vi "Build Tree.vi"(8 "Actual Path":path[](array[path]), 10 "Expected Path":path[](array[path]), 11 "Tree Refnum":refnum<vi>) -> ()   [LabVIEW 2023]
doc: "Populates the tree control identified by <B>Tree Refnum</B> with the other inputs, highlighting each row appropriately."
uses:
  11d6df90-a5f7-4652-ac9b-e2f8193509e9.vi
  <userlib>/_OpenG.lib/file/file.llb/Strip Path - Arrays__ogtk.vi
  <userlib>/_OpenG.lib/array/array.llb/Filter 1D Array with Scalar (Path)__ogtk.vi
  <userlib>/_OpenG.lib/file/file.llb/openg_file.lvlib
  <userlib>/_OpenG.lib/array/array.llb/openg_array.lvlib
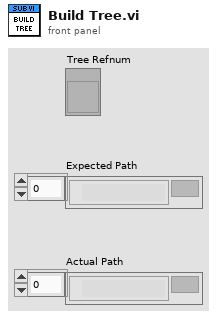
[diagram p1: front panel]
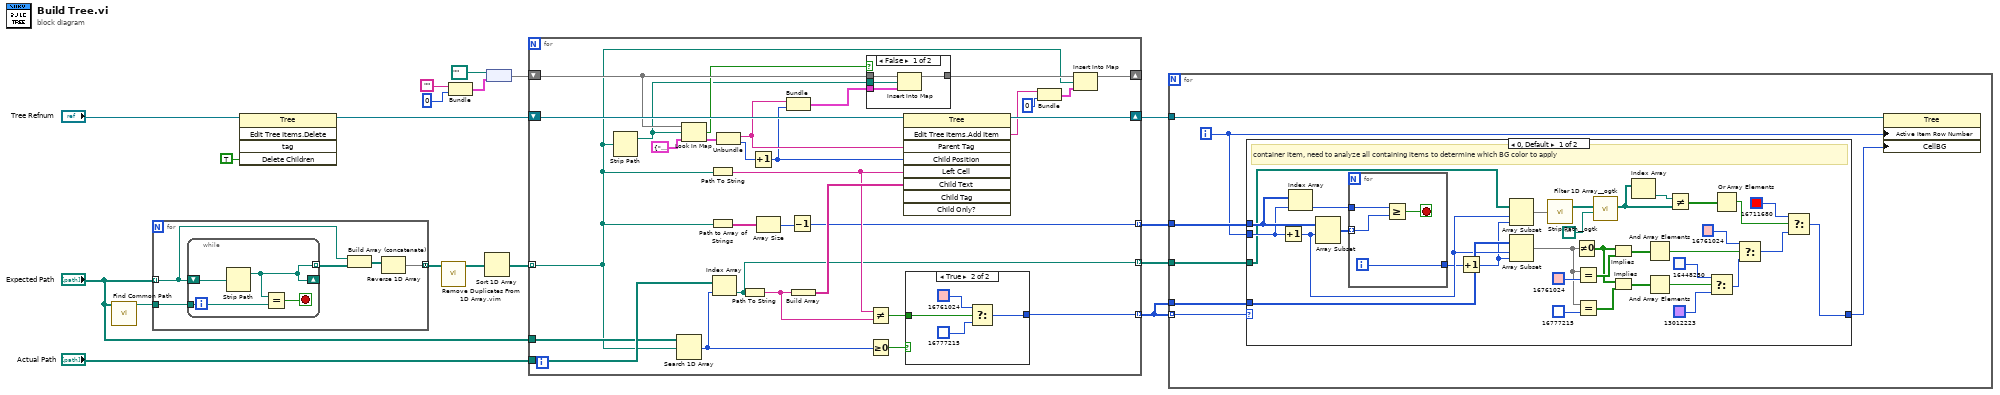
[diagram p0: block diagram]
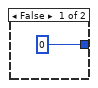
[diagram p3: hidden frame]
diagram:
  n1 = call "Find Common Path.vi"("Paths"="Expected Path") -> ("Common Path"=w7:path)  [unwired: 10 in]
  n2 = for {
    tunnel: "Expected Path" -> [w21] mode=indexing
    tunnel: [w23] -> w18 mode=concatenating
    tunnel: w7 -> [w19]
    n3 = while {
      shift-right: [w25] -> _
      shift-left: w21 -> [w27]
      tunnel: [w25] -> w22 mode=indexing
      tunnel: w19 -> [w24]
      stop <- w26 stop-if-true
      n4 = Strip Path(path=w27) -> (stripped path=w25:path)  [unwired: 1 out]
      n5 = Equal?(x=w25, y=w24) -> (x = y?=w26:bool)
    }
    n6 = Build Array (concatenate)(w21, w22) -> (w20:path[])
    n7 = Reverse 1D Array(array=w20) -> (reversed array=w23:path[])
  }
  n8 = invoke class="Tree" method="Edit Tree Items.Delete"(reference="Tree Refnum", "Delete Children"=TRUE ("Delete Children?")) -> (reference out=w12:refnum<vi>)  [unwired: 3 in, 4 out]
  n9 = call "Remove Duplicates From 1D Array.vim"("array"=w18) -> ("array with duplicates removed"=w10:path[])  [unwired: 10 in]
  n10 = Bundle("", 0) -> (w4:cluster{string, i32})  [unwired: 1 in]
  n11 = Sort 1D Array(array=w10) -> (sorted array=w2:path[])
  n12 = node(path "", w4) -> (w17:map{path, cluster{string, i32}})
  n13 = for {
    tunnel: w2 -> [w30] mode=indexing
    shift-right: [w29] -> _
    shift-left: w17 -> [w42]
    shift-right: [w56] -> w3
    shift-left: w12 -> [w57]
    tunnel: "Actual Path" -> [w55]
    tunnel: "Expected Path" -> [w54]
    tunnel: [w53] -> w9 mode=indexing
    tunnel: [w44] -> w11 mode=indexing
    tunnel: [w28] -> w1 mode=indexing
    n14 = Strip Path(path=w30) -> (stripped path=w34:path)  [unwired: 1 out]
    n15 = Search 1D Array(1D array=w54, element=w30) -> (index of element=w47:i32)  [unwired: 1 in]
    n16 = Look In Map(map=w42, key=w34, default value=cluster{string, i32} {"", -1}) -> (key not found?=w36:bool, value=w43:cluster{string, i32})
    n17 = Path To String(path=w30) -> (string=w49:string)
    n18 = Path to Array of Strings(0:w30) -> (2:w51:string[])  [unwired: 1 out]
    n19 = Index Array(array=w55, index=w47) -> (element=w28:path)
    n20 = Unbundle(w43) -> (w38:string, w39:i32)
    n21 = Path To String(path=w28) -> (string=w48:string)
    n22 = Increment(x=w39) -> (x+1=w37:i32)
    n23 = Array Size(array=w51) -> (size(s)=w52:i32)
    n24 = Bundle(w38, w37) -> (w35:cluster{string, i32})  [unwired: 1 in]
    n25 = Decrement(x=w52) -> (x-1=w44:i32)
    n26 = Build Array(w48) -> (w50:string[])
    n27 = case shown="False" w36 {
      tunnel: w42 -> [w61 w62]
      tunnel: [w60 w62] -> w41
      tunnel: w35 -> [w59 _]
      tunnel: w34 -> [w58 _]
      frame False {
        n28 = Insert Into Map(map in=w61, key=w58, value=w59) -> (map out=w60:map{path, cluster{string, i32}})  [unwired: 2 out]
      }
      frame True {
      }
    }
    n29 = Not Equal?(x=w49, y=w48) -> (x != y?=w46:bool)
    n30 = Greater Or Equal To 0?(x=w47) -> (x >= 0?=w45:bool)
    n31 = invoke class="Tree" method="Edit Tree Items.Add Item"(reference=w57, "Parent Tag"=w38, "Child Position"=w37, "Left Cell"=w49, "Child Text"=w50) -> (reference out=w56:refnum<vi>, "Edit Tree Items:Add Item"=w33:string)  [unwired: 4 in, 7 out]
    n32 = case shown="True" w45 {
      tunnel: [u32 0 w67] -> w53
      tunnel: w46 -> [_ w64]
      frame False {
      }
      frame True {
        n33 = Select(t=u32 16761024, s=w64, f=u32 16777215) -> (s? t:f=w67:u32)
      }
    }
    n34 = Bundle("Edit Tree Items:Add Item"=w33, 0) -> (w31:cluster{"Edit Tree Items:Add Item":string, i32})  [unwired: 1 in]
    n35 = Insert Into Map(map in=w41, key=w30, value=w31) -> (map out=w29:map{path, cluster{string, i32}})  [unwired: 2 out]
  }
  n36 = for {
    tunnel: w3 -> [w74]
    tunnel: w9 -> [w73] mode=indexing
    tunnel: w11 -> [w72]
    tunnel: w9 -> [w69]
    tunnel: w1 -> [w68]
    i -> [w71]
    n37 = case shown="0, Default" w73 {
      selector: w73 -> [_ w112]
      tunnel: w72 -> [w106 _]
      tunnel: w71 -> [w105 _]
      tunnel: [w81 w112] -> w70
      tunnel: w69 -> [w103 _]
      tunnel: w68 -> [w87 _]
      frame 0, Default {
        # "container item, need to analyze all containing items to determine which BG color to apply"
        n38 = Increment(x=w105) -> (x+1=w85:i32)
        n39 = Index Array(array=w106, index=w105) -> (element=w104:i32)
        n40 = Array Subset(array=w106, index=w85) -> (w107:i32[])  [unwired: 1 in]
        n41 = for {
          tunnel: w107 -> [w108] mode=indexing
          tunnel: w104 -> [w111]
          tunnel: [w109] -> w84
          i -> [w109]
          stop <- w110 stop-if-true
          n42 = Greater Or Equal?(x=w111, y=w108) -> (x >= y?=w110:bool)
        }
        n43 = Increment(x=w84) -> (x+1=w80:i32)
        n44 = Array Subset(array=w87, index=w85, length=w80) -> (w86:path[])
        n45 = Array Subset(array=w103, index=w85, length=w80) -> (w98:u32[])
        n46 = call-poly <userlib>:"Strip Path__ogtk.vi"("path"=w86) -> ("stripped path"=w79:path[])  [unwired: 1 out]
        n47 = Not Equal To 0?(x=w98) -> (x != 0?=w83:bool[])
        n48 = Equal?(x=w98, y=u32 16761024) -> (x = y?=w101:bool[])
        n49 = Equal?(x=w98, y=u32 16777215) -> (x = y?=w99:bool[])
        n50 = call-poly <userlib>:"Filter 1D Array__ogtk.vi"("items to filter"=path "", "array"=w79) -> ("filtered array"=w76:path[])  [unwired: 4 in, 1 out]
        n51 = Implies(1:w101, 2:w83) -> (0:w97:bool[])
        n52 = Implies(1:w99, 2:w83) -> (0:w96:bool[])
        n53 = Index Array(array=w76) -> (element=w77:path)  [unwired: 1 in]
        n54 = And Array Elements(Boolean array=w97) -> (logical AND=w95:bool)
        n55 = And Array Elements(Boolean array=w96) -> (logical AND=w92:bool)
        n56 = Not Equal?(x=w77, y=w76) -> (x != y?=w75:bool[])
        n57 = Select(t=u32 16448250, s=w92, f=u32 13012223) -> (s? t:f=w91:u32)
        n58 = Or Array Elements(Boolean array=w75) -> (logical OR=w82:bool)
        n59 = Select(t=u32 16761024, s=w95, f=w91) -> (s? t:f=w88:u32)
        n60 = Select(t=u32 16711680, s=w82, f=w88) -> (s? t:f=w81:u32)
      }
      frame 1.. {
        # "not a container item, apply BG color determined in previous loop"
      }
    }
    n61 = property class="Tree"(reference=w74, "Active Item Row Number"=w71, "CellBG"=w70) -> ()  [unwired: 1 in, 2 out]
  }
